vi "Digital Tach Timing.vi"(4 "time length":dbl format="%.2f", 5 "counter task type":enum16{"period measurement", "event counting"}(ring)=enum."event counting", 6 "counter timebase [Hz]":dbl=20000000.0 format="%.0p", 7 "tach counts":u32[](array[numeric])) -> (1 "number of pulses":i32, 3 "pulse positions [s]":dbl[](array[numeric]) format="%.2f")   [LabVIEW 2017]
doc: "Times the tachometer signal acquired by a digital counter."
panel:
  # "Digital Tach Timing"
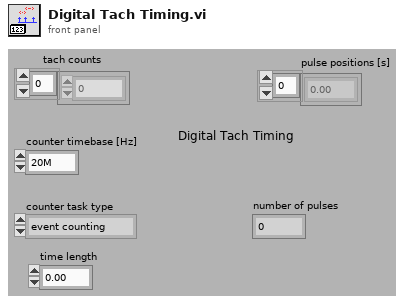
[diagram p1: front panel]
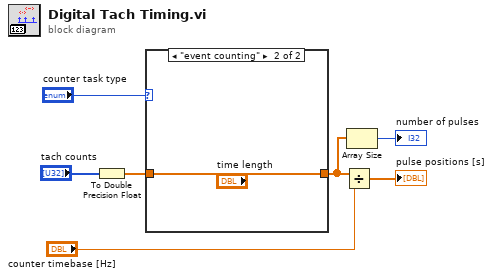
[diagram p0: block diagram]
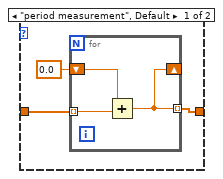
[diagram p2: hidden frame]
diagram:
  n1 = To Double Precision Float(number="tach counts") -> (double precision float=w3:dbl[])
  n2 = case shown="\"event counting\"" "counter task type" {
    tunnel: w3 -> [w9 w14]
    tunnel: [w8 w14] -> w1
    frame "period measurement", Default {
      n3 = for {
        tunnel: w9 -> [w13] mode=indexing
        shift-right: [w11] -> _
        shift-left: 0.0 -> [w12]
        tunnel: [w11] -> w8 mode=indexing
        n4 = Add(x=w12, y=w13) -> (x+y=w11:dbl)
      }
    }
    frame "event counting" {
    }
  }
  n5 = Divide(x=w1, y="counter timebase [Hz]") -> (x/y=→"pulse positions [s]":dbl[])
  n6 = Array Size(array=w1) -> (size(s)=→"number of pulses":i32)
